vi "Frequency and Value Arrays to Cluster Array.vi"(10 "Value":dbl[](array[numeric]), 11 "Frequency":dbl[](array[numeric])) -> (3 "Cluster Array":cluster{"Frequency":dbl, "Value":dbl}[](array[cluster]))   [LabVIEW 2023, in "FPT NoiseFigure UI.lvlib"]
uses:
  FPT NoiseFigure UI.lvlib
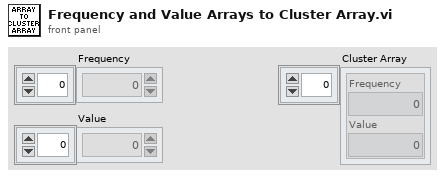
[diagram p1: front panel]
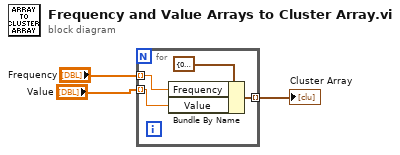
[diagram p0: block diagram]
diagram:
  n1 = for {
    tunnel: "Frequency" -> [w6] mode=indexing
    tunnel: "Value" -> [w5] mode=indexing
    tunnel: [w4] -> w3 mode=indexing
    n2 = Bundle By Name(cluster=cluster{"Frequency":dbl, "Value":dbl} {"Frequency"=0.0, "Value"=0.0} ("ENR"), "Frequency"=w6, "Value"=w5) -> (w4:cluster{"Frequency":dbl, "Value":dbl})
  }
  "Cluster Array" <- w3
